vi "Set HOST Serial Port Parameters.vi"(0 "VISA resource name":refnum<visa-resource-name>, 1 "Interface (0: Terminal)":u32(ring) items=["Terminal", "Computer"], 2 "Baud Rate (9600)":u32=9600, 5 "Flow Control (0: Xon/Xoff)":u32(ring) items=["Xon/Xoff", "None", "Rts/Cts"], 7 "Number Data Bits (1: 8 bits)":u32(ring)=1 items=["7 bits", "8 bits"], 9 "Number Stop Bits (0: 1 bit)":u32(ring) items=["1 bit", "2 bits"], 11 "error in (no error)":errorcluster, 12 "Parity (0: None)":u32(ring) items=["None", "Odd", "Even", "Ignore"], 13 "End of Line Char (2: Carriage Return/Line Feed)":u32(ring)=2 items=["Carriage Return", "Line Feed", "Carriage Return/Line Feed"]) -> (4 "VISA resource name out":refnum<visa-resource-name>, 15 "error out":errorcluster)   [LabVIEW 2013, in "Fluke 5XXX Series Multicalibrators.lvlib"]
doc: "This VI Sets the RS-232-C settings for the Calibrator rear panel SERIAL 1 FROM HOST serial port, which is saved in the Calibrator non-volatile memory. (While saving configuration data in the non-volatile memory, a period of about 2 seconds, the Calibrator does not respond to remote commands.)"
uses:
  Fluke 5XXX Series Multicalibrators.lvlib
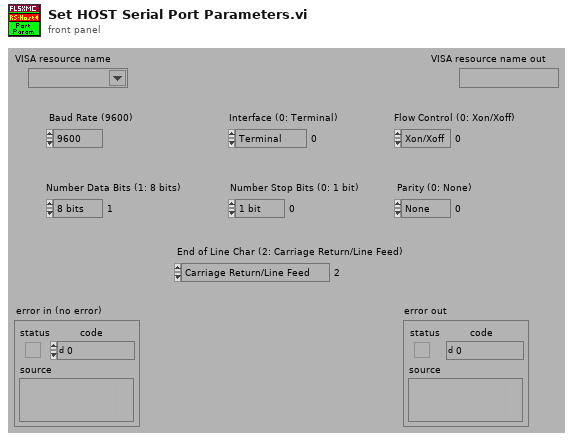
[diagram p1: front panel]
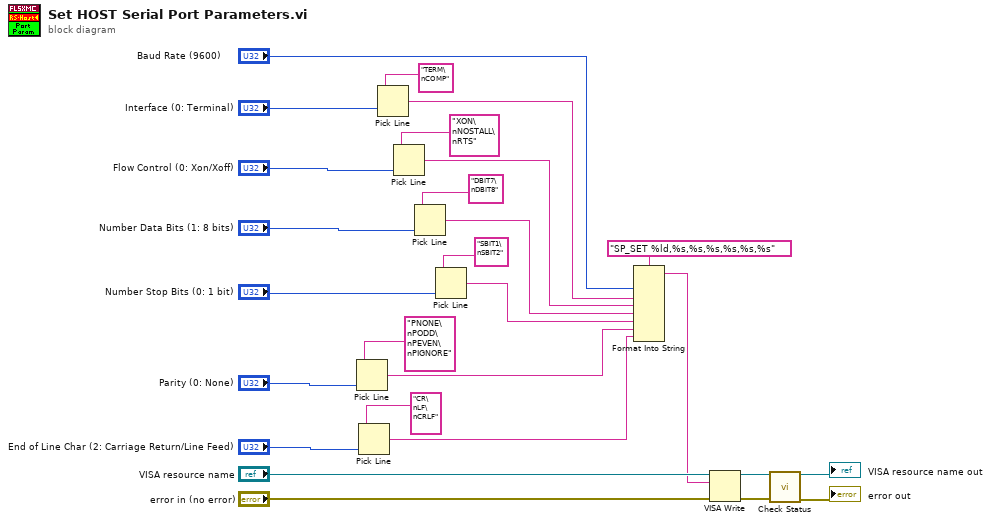
[diagram p0: block diagram]
diagram:
  n1 = Pick Line(multi-line string="PNONE\nPODD\nPEVEN\nPIGNORE" ("Reset Command"), line index="Parity (0: None)") -> (output string=w6:string)  [unwired: 1 in]
  n2 = Pick Line(multi-line string="CR\nLF\nCRLF" ("Reset Command"), line index="End of Line Char (2: Carriage Return/Line Feed)") -> (output string=w3:string)  [unwired: 1 in]
  n3 = Pick Line(multi-line string="TERM\nCOMP" ("Reset Command"), line index="Interface (0: Terminal)") -> (output string=w18:string)  [unwired: 1 in]
  n4 = Pick Line(multi-line string="XON\nNOSTALL\nRTS" ("Reset Command"), line index="Flow Control (0: Xon/Xoff)") -> (output string=w15:string)  [unwired: 1 in]
  n5 = Pick Line(multi-line string="DBIT7\nDBIT8" ("Reset Command"), line index="Number Data Bits (1: 8 bits)") -> (output string=w11:string)  [unwired: 1 in]
  n6 = Pick Line(multi-line string="SBIT1\nSBIT2" ("Reset Command"), line index="Number Stop Bits (0: 1 bit)") -> (output string=w8:string)  [unwired: 1 in]
  n7 = Format Into String(format string="SP_SET %ld,%s,%s,%s,%s,%s,%s" ("Reset Command"), "Baud Rate (9600)", w18, w15, w11, w8, w6, w3) -> (resulting string=w20:string)  [unwired: 2 in, 1 out]
  n8 = VISA Write(VISA resource name="VISA resource name", write buffer=w20, error in (no error)="error in (no error)") -> (VISA resource name out=w27:refnum<visa-resource-name>, error out=w26:errorcluster)  [unwired: 1 out]
  n9 = call "Check Status.vi"("VISA resource name"=w27, "error in (no error)"=w26) -> ("VISA resource name out"=→"VISA resource name out":refnum<visa-resource-name>, "error out"=→"error out":errorcluster)  [unwired: 12 in]
